vi "set Packet Timeout M Sec.vi"(8 "error in (no error)":errorcluster, 10 "msec":dbl, 11 "port_num":i32) -> (0 "error out":errorcluster)   [LabVIEW 2018, in "labview.lvlib"]
doc: "WINDECLSPEC void setPacketTimeoutMSec (int port_num, double msec);"
uses:
  labview.lvlib
  dxl_x86_c.dll
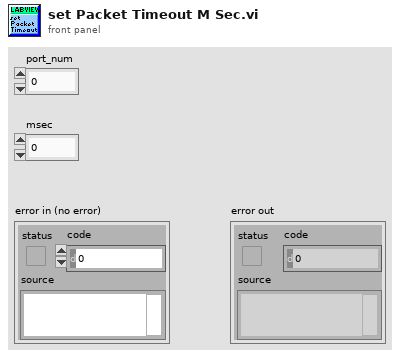
[diagram p1: front panel]
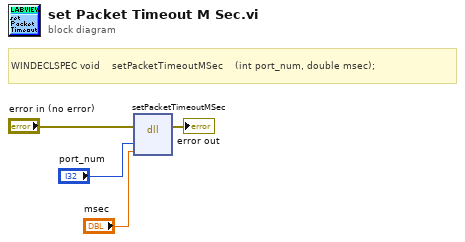
[diagram p0: block diagram]
diagram:
  # "WINDECLSPEC void    setPacketTimeoutMSec    (int port_num, double msec);"
  n1 = dll-call lib="C:/Users/joaos/OneDrive/Documents/[PhD]/Project Omnidirectional Vehicle/Vanes/LabView_code/joaoandthethreestands/DynamixelSDK-3.7.31/labview/new_compilation/dxl_x86_c.*" fn="setPacketTimeoutMSec"(error in="error in (no error)", "port_num"="port_num", "msec"="msec") -> (error out=→"error out":errorcluster)  [unwired: 5 in, 1 out]
